vi "Find Header Value - Multiple.vi"(7 "Header":string, 8 "error in (no error)":errorcluster, 10 "headers":T1[](array[typedef])) -> (0 "error out":errorcluster, 1 "Found?":bool, 2 "Values":string[](array[string]))   [LabVIEW 2020, in "Blue Easy HTTP OpenSource.lvlib"]
doc: "Finds the value of a specific Header from a list of HTTP headers and values.\n\nThe Header input is not case sensitive."
uses:
  Blue Easy HTTP OpenSource.lvlib
  HTTP Header.ctl
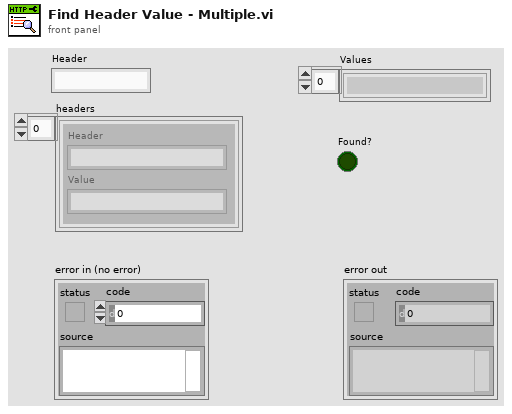
[diagram p1: front panel]
types:
  T1 = typedef "Blue Easy HTTP OpenSource.lvlib/HTTP Header.ctl" = cluster{"Header":string, "Value":string}
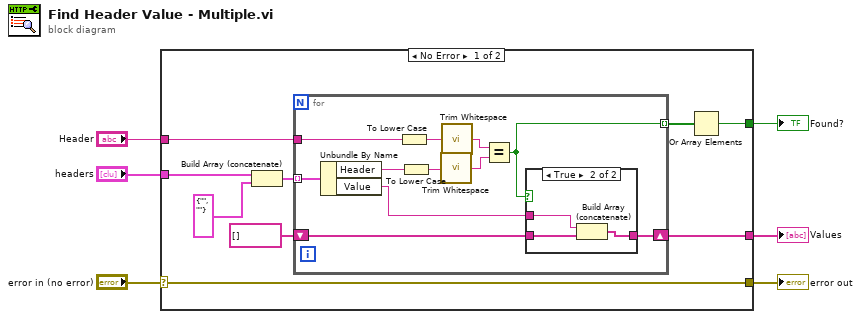
[diagram p0: block diagram]
diagram:
  n1 = case shown="No Error" "error in (no error)" {
    selector: "error in (no error)" -> [w15 w31]
    tunnel: [w15 w31] -> w5
    tunnel: "headers" -> [w10 _]
    tunnel: [w9 _] -> w3
    tunnel: [w8 _] -> w2
    tunnel: "Header" -> [w7 _]
    frame No Error {
      n2 = Build Array (concatenate)(w10, T1 {"Header"="", "Value"=""} ("HTTP Header")) -> (w13:T1[])
      n3 = for {
        tunnel: [w20] -> w11 mode=indexing
        tunnel: w13 -> [w22] mode=indexing
        shift-right: [w17] -> w8
        shift-left: string[] [] -> [w19]
        tunnel: w7 -> [w16]
        n4 = Unbundle By Name(w22) -> ("Header"=w21:string, "Value"=w18:string)
        n5 = To Lower Case(string=w16) -> (all lower case string=w25:string)
        n6 = To Lower Case(string=w21) -> (all lower case string=w26:string)
        n7 = call <vilib>:"Trim Whitespace.vi"("string"=w26) -> ("trimmed string"=w23:string)  [unwired: 1 in]
        n8 = call <vilib>:"Trim Whitespace.vi"("string"=w25) -> ("trimmed string"=w24:string)  [unwired: 1 in]
        n9 = Equal?(x=w24, y=w23) -> (x = y?=w20:bool)
        n10 = case shown="True" w20 {
          tunnel: w19 -> [w27 w30]
          tunnel: w18 -> [_ w29]
          tunnel: [w27 w28] -> w17
          frame False {
          }
          frame True {
            n11 = Build Array (concatenate)(w29, w30) -> (w28:string[])
          }
        }
      }
      n12 = Or Array Elements(Boolean array=w11) -> (logical OR=w9:bool)
    }
    frame Error {
    }
  }
  "error out" <- w5
  "Found?" <- w3
  "Values" <- w2
